vi "Update.vi"(8 "error in (no error)":errorcluster, 10 "Message in":refnum<class "UpdateMessage.lvclass">, 11 "Galvo in":refnum<class "ImagingModeSPIM.lvclass">) -> (0 "error out":errorcluster, 3 "Galvo out":refnum<class "ImagingModeSPIM.lvclass">)   [LabVIEW 2012, in "ImagingModeSPIM.lvclass"]
doc: "The update method processes the command 'update'. \n\nThe command 'update' is used for receiving new values to be set to the private data of the class. This could be seen as a public set method for setting new parameters to the private class data."
uses:
  ImagingModeSPIM.lvclass
  <vilib>/Distrio/Murmex/UpdateMessage/UpdateMessage.lvclass
  ImagingModeSPIM.lvclass/ImagingModeSPIM.ctl
  Controls/waveform_enum.ctl
  <vilib>/Distrio/Murmex/Murmex/Murmex.lvclass
panel:
  # "This method is called when the UPDATE\ntrigger is sent. \n\nOverride this method when your component needs to\nrespond to this trigger. \n\nCall parent for proper implementation"
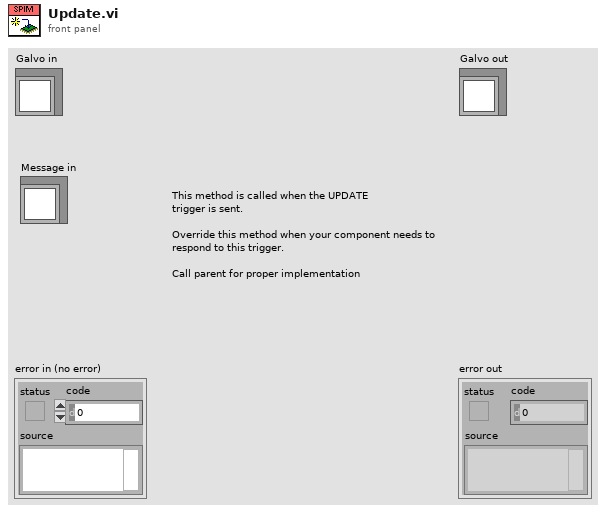
[diagram p1: front panel]
types:
  T1 = typedef "ImagingModeSPIM.lvclass/waveform_enum.ctl" = enum16{"triangular", "sawtooth", "sinusodial"}
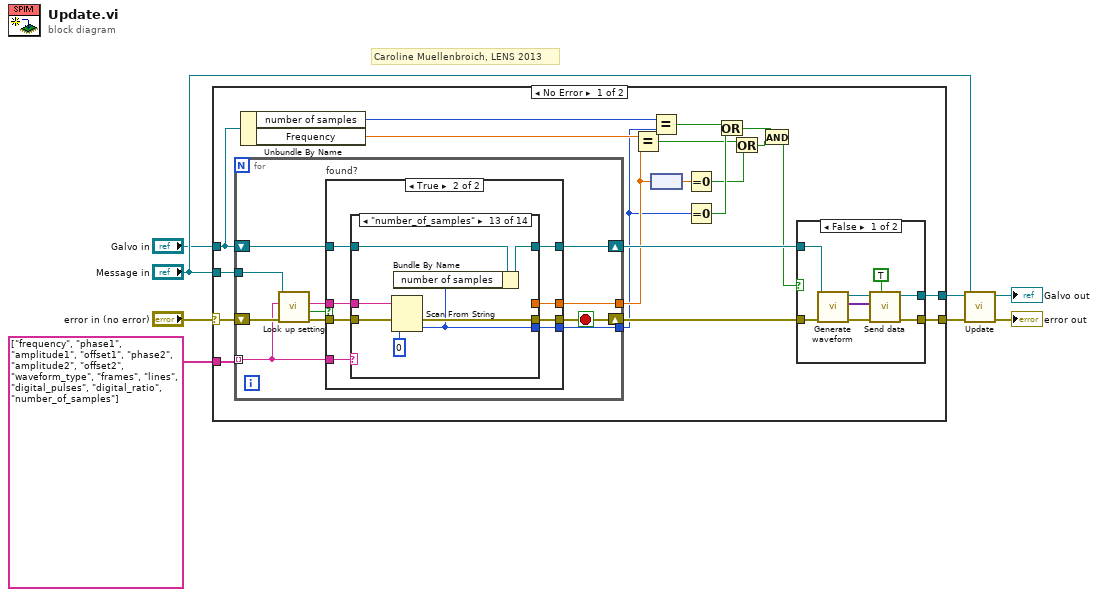
[diagram p0: block diagram]
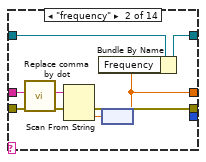
[diagram p5: hidden frame]
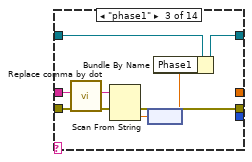
[diagram p6: hidden frame]
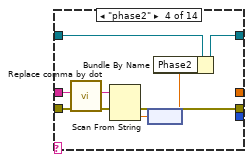
[diagram p7: hidden frame]
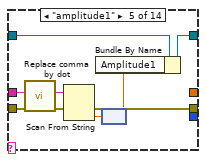
[diagram p8: hidden frame]
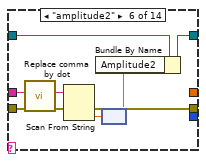
[diagram p9: hidden frame]
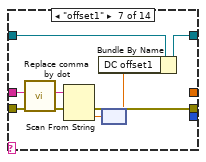
[diagram p10: hidden frame]
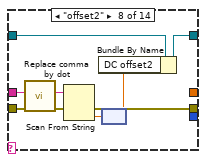
[diagram p11: hidden frame]
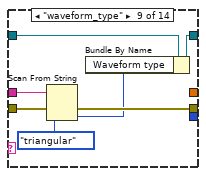
[diagram p12: hidden frame]
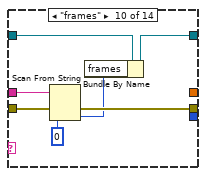
[diagram p13: hidden frame]
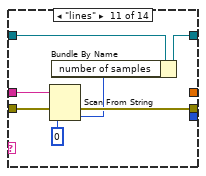
[diagram p14: hidden frame]
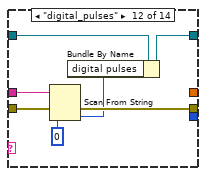
[diagram p15: hidden frame]
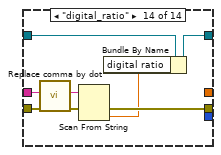
[diagram p16: hidden frame]
diagram:
  # "Caroline Muellenbroich, LENS 2013"
  n1 = case shown="No Error" "error in (no error)" {
    selector: "error in (no error)" -> [w28 w160]
    tunnel: [w23 w161] -> w5
    tunnel: "Galvo in" -> [w21 w161]
    tunnel: [w22 w160] -> w4
    tunnel: "Message in" -> [w27 _]
    tunnel: string[] ["frequency", "phase1", "amplitude1", "offset1", "phase2", "amplitude2", "offset2", "waveform_type", "frames", "lines", "digital_pulses", "digital_ratio", "number_of_samples"] ("key chains") -> [w24 _]
    frame No Error {
      n2 = for {
        tunnel: w27 -> [w48]
        tunnel: w24 -> [w42] mode=indexing
        shift-right: [w41] -> w26
        shift-left: w28 -> [w49]
        shift-right: [w44] -> w25
        shift-left: w21 -> [w45]
        tunnel: [w40] -> w19
        tunnel: [w39] -> w16
        stop <- w41 stop-if-true
        n3 = call <vilib>:"Look up setting.vi"("error in (no error)"=w49, "tag name"=w42, "UpdateMessage in"=w48) -> ("error out"=w46:errorcluster, "found?"=w47:bool, "value"=w43:string)  [unwired: 5 in, 1 out]
        n4 = case "found?" shown="True" w47 {
          tunnel: w46 -> [w51 w56]
          tunnel: [w51 w57] -> w41
          tunnel: w45 -> [w50 w54]
          tunnel: [w50 w55] -> w44
          tunnel: w43 -> [_ w59]
          tunnel: w42 -> [_ w58]
          tunnel: [_ w53] -> w40
          tunnel: [_ w52] -> w39
          frame False {
          }
          frame True {
            n5 = case shown="\"number_of_samples\"" w58 {
              tunnel: w59 -> [_ w68 w76 w84 w92 w100 w108 w116 w121 w127 w134 w141 w148 w158]
              tunnel: [w61 w66 w74 w82 w90 w98 w106 w114 w120 w128 w135 w142 w149 w156] -> w57
              tunnel: w56 -> [w61 w69 w77 w85 w93 w101 w109 w117 w122 w129 w136 w143 w150 w159]
              tunnel: [w60 w64 w71 w79 w87 w95 w103 w111 w123 w130 w137 w144 w151 w155] -> w55
              tunnel: w54 -> [w60 w67 w75 w83 w91 w99 w107 w115 w124 w131 w138 w145 w152 w157]
              tunnel: [_ w62 _ _ _ _ _ _ _ _ _ _ _ _] -> w53
              tunnel: [_ _ _ _ _ _ _ _ _ _ _ _ w146 _] -> w52
              frame Default {
              }
              frame "frequency" {
                n6 = call <vilib>:"Replace comma by dot.vi"("input string"=w68) -> ("result string"=w63:string)  [unwired: 10 in]
                n7 = Scan From String(input string=w63, error in=w69) -> (error out=w66:errorcluster, output 1=w65:dbl)  [unwired: 3 in, 2 out]
                n8 = node(w65) -> (w62:dbl[unit])
                n9 = Bundle By Name(cluster=w67, "Frequency"=w62) -> (w64:refnum<class "ImagingModeSPIM.lvclass">)
              }
              frame "phase1" {
                n10 = call <vilib>:"Replace comma by dot.vi"("input string"=w76) -> ("result string"=w70:string)  [unwired: 10 in]
                n11 = Scan From String(input string=w70, error in=w77) -> (error out=w74:errorcluster, output 1=w73:dbl)  [unwired: 3 in, 2 out]
                n12 = node(w73) -> (w72:dbl[unit])
                n13 = Bundle By Name(cluster=w75, "Phase1"=w72) -> (w71:refnum<class "ImagingModeSPIM.lvclass">)
              }
              frame "phase2" {
                n14 = call <vilib>:"Replace comma by dot.vi"("input string"=w84) -> ("result string"=w78:string)  [unwired: 10 in]
                n15 = Scan From String(input string=w78, error in=w85) -> (error out=w82:errorcluster, output 1=w81:dbl)  [unwired: 3 in, 2 out]
                n16 = node(w81) -> (w80:dbl[unit])
                n17 = Bundle By Name(cluster=w83, "Phase2"=w80) -> (w79:refnum<class "ImagingModeSPIM.lvclass">)
              }
              frame "amplitude1" {
                n18 = call <vilib>:"Replace comma by dot.vi"("input string"=w92) -> ("result string"=w86:string)  [unwired: 10 in]
                n19 = Scan From String(input string=w86, error in=w93) -> (error out=w90:errorcluster, output 1=w89:dbl)  [unwired: 3 in, 2 out]
                n20 = node(w89) -> (w88:dbl[unit])
                n21 = Bundle By Name(cluster=w91, "Amplitude1"=w88) -> (w87:refnum<class "ImagingModeSPIM.lvclass">)
              }
              frame "amplitude2" {
                n22 = call <vilib>:"Replace comma by dot.vi"("input string"=w100) -> ("result string"=w94:string)  [unwired: 10 in]
                n23 = Scan From String(input string=w94, error in=w101) -> (error out=w98:errorcluster, output 1=w97:dbl)  [unwired: 3 in, 2 out]
                n24 = node(w97) -> (w96:dbl[unit])
                n25 = Bundle By Name(cluster=w99, "Amplitude2"=w96) -> (w95:refnum<class "ImagingModeSPIM.lvclass">)
              }
              frame "offset1" {
                n26 = call <vilib>:"Replace comma by dot.vi"("input string"=w108) -> ("result string"=w102:string)  [unwired: 10 in]
                n27 = Scan From String(input string=w102, error in=w109) -> (error out=w106:errorcluster, output 1=w105:dbl)  [unwired: 3 in, 2 out]
                n28 = node(w105) -> (w104:dbl[unit])
                n29 = Bundle By Name(cluster=w107, "DC offset1"=w104) -> (w103:refnum<class "ImagingModeSPIM.lvclass">)
              }
              frame "offset2" {
                n30 = call <vilib>:"Replace comma by dot.vi"("input string"=w116) -> ("result string"=w110:string)  [unwired: 10 in]
                n31 = Scan From String(input string=w110, error in=w117) -> (error out=w114:errorcluster, output 1=w113:dbl)  [unwired: 3 in, 2 out]
                n32 = node(w113) -> (w112:dbl[unit])
                n33 = Bundle By Name(cluster=w115, "DC offset2"=w112) -> (w111:refnum<class "ImagingModeSPIM.lvclass">)
              }
              frame "waveform_type" {
                n34 = Scan From String(input string=w121, error in=w122, default 1=waveform_enum."triangular" ("Waveform type")) -> (error out=w120:errorcluster, output 1=w118:T1)  [unwired: 2 in, 2 out]
                n35 = Bundle By Name(cluster=w124, "Waveform type"=w118) -> (w123:refnum<class "ImagingModeSPIM.lvclass">)
              }
              frame "frames" {
                n36 = Scan From String(input string=w127, error in=w129, default 1=0) -> (error out=w128:errorcluster, output 1=w125:i32)  [unwired: 2 in, 2 out]
                n37 = Bundle By Name(cluster=w131, "frames"=w125) -> (w130:refnum<class "ImagingModeSPIM.lvclass">)
              }
              frame "lines" {
                n38 = Scan From String(input string=w134, error in=w136, default 1=0) -> (error out=w135:errorcluster, output 1=w132:i32)  [unwired: 2 in, 2 out]
                n39 = Bundle By Name(cluster=w138, "number of samples"=w132) -> (w137:refnum<class "ImagingModeSPIM.lvclass">)
              }
              frame "digital_pulses" {
                n40 = Scan From String(input string=w141, error in=w143, default 1=0) -> (error out=w142:errorcluster, output 1=w139:i32)  [unwired: 2 in, 2 out]
                n41 = Bundle By Name(cluster=w145, "digital pulses"=w139) -> (w144:refnum<class "ImagingModeSPIM.lvclass">)
              }
              frame "number_of_samples" {
                n42 = Scan From String(input string=w148, error in=w150, default 1=0) -> (error out=w149:errorcluster, output 1=w146:i32)  [unwired: 2 in, 2 out]
                n43 = Bundle By Name(cluster=w152, "number of samples"=w146) -> (w151:refnum<class "ImagingModeSPIM.lvclass">)
              }
              frame "digital_ratio" {
                n44 = call <vilib>:"Replace comma by dot.vi"("input string"=w158) -> ("result string"=w154:string)  [unwired: 10 in]
                n45 = Scan From String(input string=w154, error in=w159) -> (error out=w156:errorcluster, output 1=w153:dbl)  [unwired: 3 in, 2 out]
                n46 = Bundle By Name(cluster=w157, "digital ratio"=w153) -> (w155:refnum<class "ImagingModeSPIM.lvclass">)
              }
            }
          }
        }
      }
      n47 = Unbundle By Name(w21) -> ("number of samples"=w18:i32, "Frequency"=w20:dbl[unit])
      n48 = Equal?(x=w20, y=w19) -> (x = y?=w12:bool)
      n49 = Equal?(x=w18, y=w16) -> (x = y?=w15:bool)
      n50 = node(w19) -> (w17:dbl)
      n51 = Equal To 0?(x=w17) -> (x = 0?=w13:bool)
      n52 = Equal To 0?(x=w16) -> (x = 0?=w14:bool)
      n53 = Or(x=w15, y=w14) -> (x .or. y?=w10:bool)
      n54 = Or(x=w12, y=w13) -> (x .or. y?=w11:bool)
      n55 = And(x=w10, y=w11) -> (x .and. y?=w9:bool)
      n56 = case shown="False" w9 {
        tunnel: w26 -> [w35 w38]
        tunnel: w25 -> [w33 w37]
        tunnel: [w30 w37] -> w23
        tunnel: [w29 w38] -> w22
        frame False {
          n57 = call-dynamic "Generate waveform.vi"("error in (no error)"=w35, "Galvo in"=w33) -> ("error out"=w34:errorcluster, "Array"=w31:variant[], "Galvo out"=w32:refnum<class "ImagingModeSPIM.lvclass">)  [unwired: 7 in]
          n58 = call <vilib>:"Send data.vi"("is finalised data? (T)"=TRUE, "error in (no error)"=w34, "data (channels array)"=w31, "Murmex in"=w32) -> ("error out"=w29:errorcluster, "Murmex out"=w30:refnum<class "ImagingModeSPIM.lvclass">)  [unwired: 6 in]
        }
        frame True {
        }
      }
    }
    frame Error {
    }
  }
  n59 = call-parent "Update.vi"("error in (no error)"=w4, "Message in"="Message in", "Murmex in"=w5) -> ("error out"=→"error out":errorcluster, "Murmex out"=→"Galvo out":refnum<class "ImagingModeSPIM.lvclass">)  [unwired: 7 in]
